vi "Convert String To Boolean.vi"(8 "error in (no error)":errorcluster, 10 "Value":string, 11 "Bool Refnum":refnum<vi>) -> (0 "error out":errorcluster)   [LabVIEW 2013]
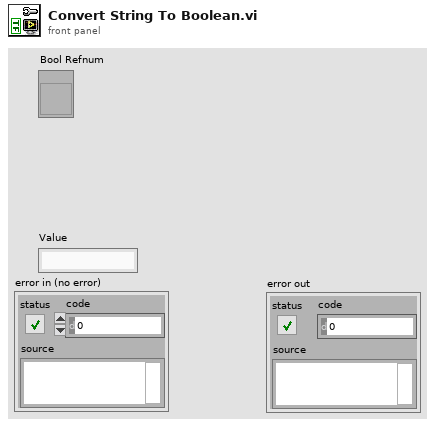
[diagram p1: front panel]
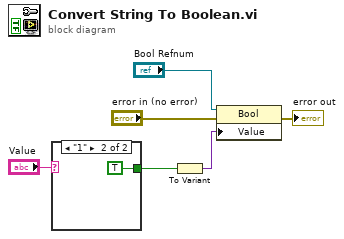
[diagram p0: block diagram]
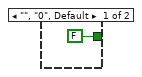
[diagram p2: hidden frame]
diagram:
  n1 = case shown="\"1\"" "Value" {
    tunnel: [FALSE TRUE] -> w6
    frame "", "0", Default {
    }
    frame "1" {
    }
  }
  n2 = To Variant(anything=w6) -> (Variant=w2:variant)
  n3 = property class="Bool"(reference="Bool Refnum", error in="error in (no error)", "Value"=w2) -> (error out=→"error out":errorcluster)  [unwired: 1 out]
